vi "EOL Printing.vi"(6 "Print?":bool, 8 "error in (no error)":errorcluster, 9 "DATA":string="E159914\n181120SD\n00001", 11 "Path":path=path "D:/Valeo/Micriphone Test/UI/ME79.btw") -> (0 "error out":errorcluster)   [LabVIEW 2018]
panel:
  in  "BarTender.IBtApplication":refnum<k7>
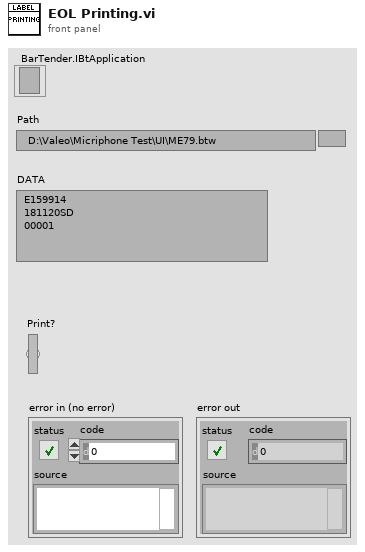
[diagram p1: front panel]
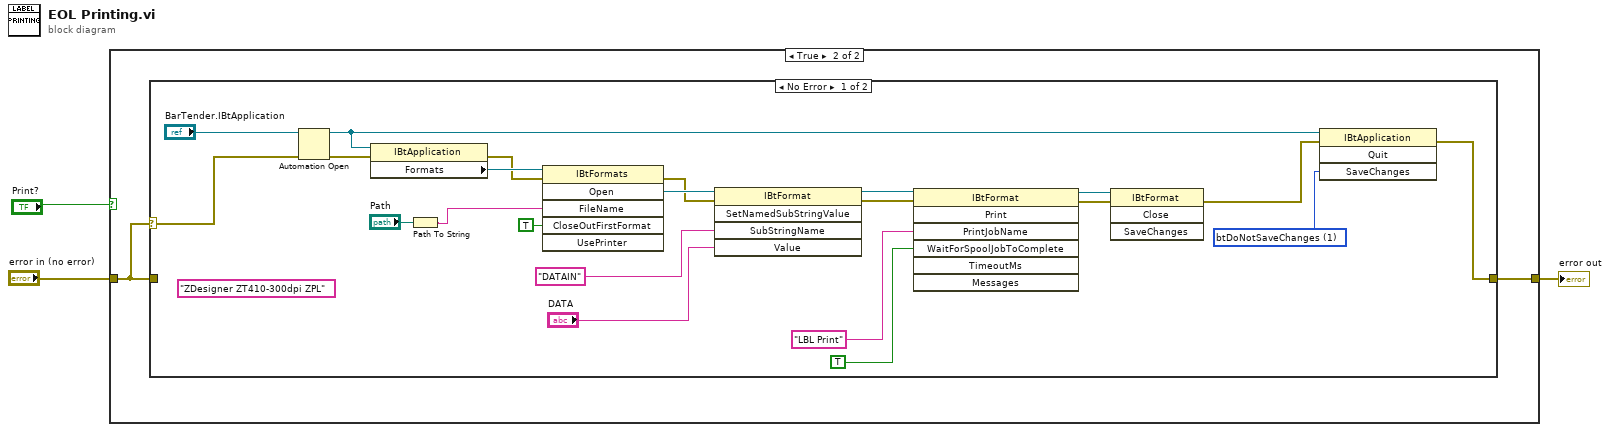
[diagram p0: block diagram]
diagram:
  n1 = case shown="True" "Print?" {
    tunnel: "error in (no error)" -> [w4 w5]
    tunnel: [w4 w6] -> w1
    frame False {
    }
    frame True {
      n2 = case shown="No Error" w5 {
        selector: w5 -> [w7 _]
        tunnel: [w8 w29] -> w6
        tunnel: w5 -> [_ w29]
        frame No Error {
          (unwired) "ZDesigner ZT410-300dpi ZPL" ("UsePrinter")
          w20 = 1 items=["btPromptSave", "btDoNotSaveChanges", "btSaveChanges"] ("SaveChanges")
          n3 = Automation Open(error in (no error)=w7, Automation Refnum="BarTender.IBtApplication") -> (Automation Refnum=w21:refnum<k7>, error out=w27:errorcluster)  [unwired: 2 in]
          n4 = property class="IBtApplication"(reference=w21, error in=w27) -> (error out=w25:errorcluster, "Formats"=w26:refnum<k7>)  [unwired: 1 out]
          n5 = Path To String(path="Path") -> (string=w23:string)
          n6 = invoke class="IBtFormats" method="Open"(reference=w26, error in=w25, "FileName"=w23, "CloseOutFirstFormat"=TRUE) -> (error out=w17:errorcluster, "Open"=w18:refnum<k7>)  [unwired: 2 in, 4 out]
          n7 = invoke class="IBtFormat" method="SetNamedSubStringValue"(reference=w18, error in=w17, "SubStringName"="DATAIN" ("FieldnameSampleDataList"), "Value"="DATA") -> (reference out=w15:refnum<k7>, error out=w16:errorcluster)  [unwired: 1 in, 3 out]
          n8 = invoke class="IBtFormat" method="Print"(reference=w15, error in=w16, "PrintJobName"="LBL Print", "WaitForSpoolJobToComplete"=TRUE) -> (reference out=w13:refnum<k7>, error out=w12:errorcluster)  [unwired: 3 in, 5 out]
          n9 = invoke class="IBtFormat" method="Close"(reference=w13, error in=w12) -> (error out=w11:errorcluster)  [unwired: 2 in, 3 out]
          n10 = invoke class="IBtApplication" method="Quit"(reference=w21, error in=w11, "SaveChanges"=w20) -> (error out=w8:errorcluster)  [unwired: 1 in, 3 out]
        }
        frame Error {
        }
      }
    }
  }
  "error out" <- w1
